vi "Stop Configuration VI.vi"(8 "error in (no error)":errorcluster, 10 "Subpanel Queue In":refnum<queue>, 11 "VI in":T1) -> (0 "error out":errorcluster, 2 "Subpanel Queue Out":refnum<queue>, 3 "Variant Out":variant)   [LabVIEW 2018]
doc: "Queue message stops the configuration VI."
uses:
  controls/VI Reference Type.ctl
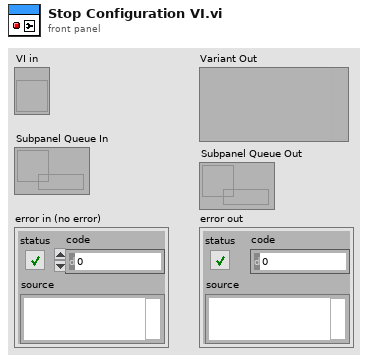
[diagram p1: front panel]
types:
  T1 = typedef "VI Reference Type.ctl" = refnum<vi>
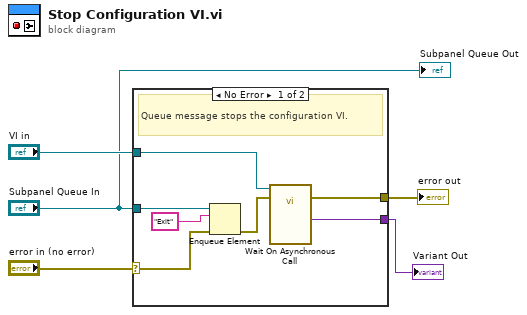
[diagram p0: block diagram]
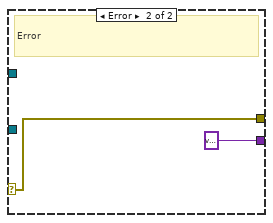
[diagram p2: hidden frame]
diagram:
  n1 = case shown="No Error" "error in (no error)" {
    selector: "error in (no error)" -> [w6 w14]
    tunnel: "Subpanel Queue In" -> [w11 _]
    tunnel: [w10 w14] -> w5
    tunnel: "VI in" -> [w8 _]
    tunnel: [w7 variant ("Variant Out")] -> w3
    frame No Error {
      # "Queue message stops the configuration VI."
      n2 = Enqueue Element(queue=w11, element="Exit", error in (no error)=w6) -> (error out=w9:errorcluster)  [unwired: 1 in, 2 out]
      n3 = call-by-ref "Wait On Asynchronous Call"(reference=w8, error in=w9) -> (error out=w10:errorcluster, "Parameters Out"=w7:variant)  [unwired: 10 in, 2 out]
    }
    frame Error {
      # "Error"
    }
  }
  "error out" <- w5
  "Variant Out" <- w3
  "Subpanel Queue Out" <- "Subpanel Queue In"
